vi "Solve2.vi"(8 "Error In":errorcluster, 11 "object in":refnum<class "2021_16.lvclass">) -> (0 "Error Out":errorcluster, 2 "Result":u64, 3 "object out":refnum<class "2021_16.lvclass">)   [LabVIEW 2020, in "2021_16.lvclass"]
uses:
  2021_16.lvclass
  2021_16.lvclass/2021_16.ctl
panel:
  out "literal value":u64
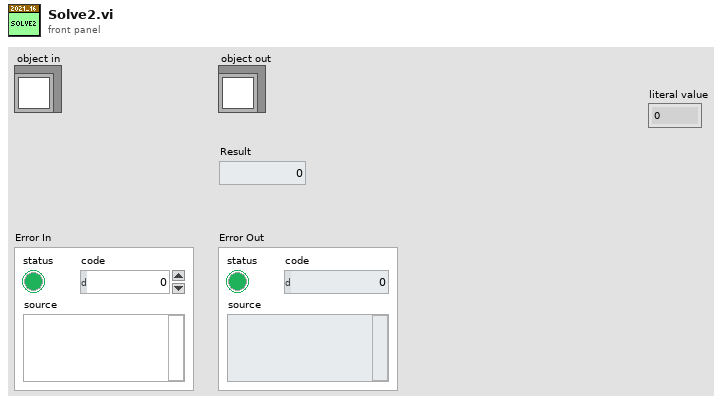
[diagram p1: front panel]
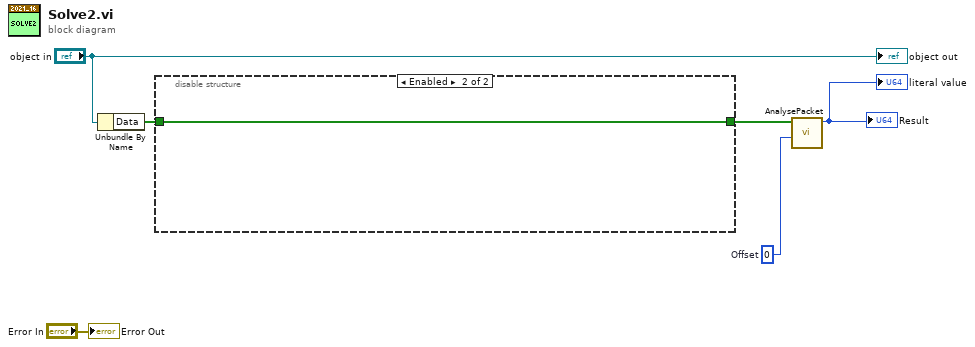
[diagram p0: block diagram]
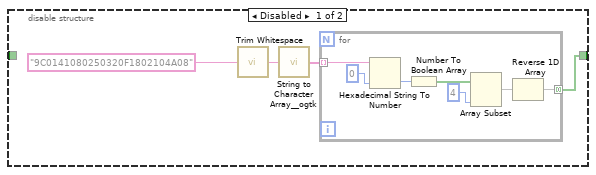
[diagram p2: hidden frame]
diagram:
  w3 = 0  # Offset
  n1 = Unbundle By Name("object in") -> ("Data"=w2:bool[])
  n2 = disable-structure shown="Enabled" {
    disable-tunnel: [w7 w18] -> w4
    disable-tunnel: w2 -> [_ w18]
    frame Disabled {
      n3 = call <vilib>:"Trim Whitespace.vi"("string"="9C0141080250320F1802104A08") -> ("trimmed string"=w10:string)  [unwired: 1 in]
      n4 = call <userlib>:"String to Character Array__ogtk.vi"("Input String"=w10) -> ("Character Array"=w9:string[])
      n5 = for {
        tunnel: w9 -> [w17] mode=indexing
        tunnel: [w11] -> w7 mode=concatenating
        n6 = Hexadecimal String To Number(string=w17, default (0uL)=u8 0 ("default (0 U32)")) -> (number=w15:u8)  [unwired: 1 in, 1 out]
        n7 = Number To Boolean Array(number=w15) -> (Boolean array=w14:bool[])
        n8 = Array Subset(array=w14, length=4) -> (w12:bool[])  [unwired: 1 in]
        n9 = Reverse 1D Array(array=w12) -> (reversed array=w11:bool[])
      }
    }
    frame Enabled {
    }
  }
  n10 = call "AnalysePacket.vi"("Offset"=w3, "Data"=w4) -> ("Result"=→"Result" →"literal value":u64)  [unwired: 7 in, 2 out]
  "Error Out" <- "Error In"
  "object out" <- "object in"
